vi "Main v1.31.vi"() -> ()   [LabVIEW 2017]
doc: "v0.85:\n- Counts for rejects and total\n\nv0.5:\n\n- Added Reject to Manual Mode\n- Send reject pallet cluster during manual mode\n- Run continuous manual happens only when no error has occured"
uses:
  Controls/Main Tabs v0.1.ctl
  Controls/Auto.ctl
  RT/Controls/Auto Delays.ctl
  RT/Controls/Auto Times.ctl
  support/Controls/General Para.ctl
  Controls/UI Data.ctl
  support/Controls/Auto Stats.ctl
  Controls/Logging FGV.ctl
  support/Message Queue/Enqueue Message (Single).vi
  GV/Maintenance GV.vi
  <vilib>/Utility/error.llb/Error Cluster From Error Code.vi
  <vilib>/ErrorRing/Error Ring.xnode
  support/Message Queue/Message Queue.lvlib
  support/User Event - Stop/User Event - Stop.lvlib
panel:
  in  "General Para 2":T1={"Max. Cons."=5.0, "Offset 1"=0.0, "Offset 2"=0.0, "Offset 3"=0.0, "Offset 4"=0.0} caption="General Para"
  in  "Auto Para 2":T2={"Agitator Delays"=[250, 350], "TF Delays"=[700, 800, 2], "Insertion Delays"=[100, 500], "Cutting Delays"=[300, 300, 100], "PF Delays"=[250, 30000], "Measur. Delays"=[500.0, 188.9, 1.0], "Reject Delays"=[500], "BF Delays"=[1000, 1000]}
  out "Shutdown?":bool
  out "Boolean 8":bool
  out "Boolean 7":bool
  out "Boolean 6":bool
  out "Boolean 5":bool
  out "Boolean 4":bool
  out "Boolean 3":bool
  out "Boolean 2":bool
  out "Boolean":bool
  in  "Reject Pallets":T3
  out "Date-Time":string caption="Dip-Tube Assembly Automation (HMI) v1.2"
  out "Main Tab":T4
  in  "All IOs":bool
  in  "Autocycle":T5
  in  "Manual":bool
  in  "Parameters":bool
  in  "Maintenance":bool
  in  "General Para":T1={"Max. Cons."=5.0, "Offset 1"=0.0, "Offset 2"=0.0, "Offset 3"=0.0, "Offset 4"=0.0} {"Offset 4" format="%.2f"; "Offset 3" format="%.2f"; "Offset 2" format="%.2f"; "Offset 1" format="%.2f"}
  in  "BF Para":cluster{"Delay 1":u32, "Delay 2":u32}={"Delay 1"=1000, "Delay 2"=1000}
  in  "Reject Para":cluster{"Delay":u32}={"Delay"=400}
  in  "Meas. Para":T6={"Delay"=500.0, "Mean Length"=188.9, "Tolerance"=1.0}
  in  "PF Para":cluster{"Delay":u32, "Timeout":u32}={"Delay"=1000, "Timeout"=1000}
  in  "Tube Feeder Para":T7={"Delay"=400, "Delay 2"=250, "Max Attempts"=250}
  in  "Cutting Para":T8={"Delay"=400, "Delay 2"=250, "Delay 3"=250}
  in  "Agitator Para":cluster{"Delay":u32, "Timeout":u32}={"Delay"=400, "Timeout"=250}
  in  "Insertion Para":cluster{"Delay 1":u32, "Delay 2":u32}={"Delay 1"=1000, "Delay 2"=1000}
  in  "Save Para":bool
  in  "Home Para":bool
  out "OEE":dbl format="%#.1f"
  out "QUA":dbl=100.0 min=0.0 max=100.0 step=0.1
  in  "Ideal Time":dbl=2.0 min=0.0 max=100.0 step=0.1
  in  "AVL":dbl=100.0 min=0.0 max=100.0 step=0.1
  out "Rejects 2":u32 caption="Rejects"
  in  "Reset MCount":bool
  in  "Enable BF?":bool
  in  "Enable Agitate?":bool
  in  "Enable Reject?":bool
  in  "Toggle Motor":bool
  in  "Continuous?":bool
  in  "Enable Measure?":bool
  in  "Enable Index?":bool
  in  "Enable PF?":bool
  in  "Manual Para":T2={"Agitator Delays"=[400, 250], "TF Delays"=[700, 800, 2], "Insertion Delays"=[100, 500], "Cutting Delays"=[300, 300, 100], "PF Delays"=[250, 30000], "Measur. Delays"=[500.0, 188.9, 1.0], "Reject Delays"=[500], "BF Delays"=[1000, 1000]}
  in  "Enable Cutting?":bool
  in  "Enable Insertion?":bool
  in  "Run Manual":bool
  in  "Enable TF?":bool
  in  "Home Manual":bool
  out "Status 2":T10
  out "Measurements":T11 {"Height 1" format="%#.2f"; "Height 2" format="%#.2f"; "Height 3" format="%#.2f"; "Height 4" format="%#.2f"}
  out "Output Count":u32 caption="Output\nCount"
  out "PRF":dbl=100.0 min=0.0 max=100.0 step=0.1
  in  "End Cycle":bool
  out "Statuses":string[][](table)
  in  "All IO":bool
  in  "Stats":bool
  in  "Home AC":bool
  out "Status":string
  out "Good":u32 format="%06.0f"
  out "Cycle Time":dbl format="%0.2f"
  out "Rejects":u32 format="%06.0f"
  out "Total Count 2":u32 caption="Total Count"
  out "Avg. Time":dbl caption="Avg. Cycle Time (s)" format="%#.3f"
  out "Output Chart":T12(graph)
  out "Reject Count":u32
  out "Good Count":u32
  out "Total Time":dbl caption="Effective Cycle Time (s)" format="%#.3f"
  out "Time Chart":T13(graph)
  out "OEE Chart":T14(graph)
  out "Timestamp":string caption="Date & Timestamp"
  out "Latest Measure.":T15 caption="Latest Measurements" {"Length 1 (mm)" format="%#.2f"}
  out "Auto Times":T9
  in  "Back Stats":bool
  out "OEE 2":T14 caption="Latest Measurements" {"AVL" format="%#.1f"; "PRF" format="%#.1f"; "QUA" format="%#.1f"; "OEE" format="%#.1f"}
  out "Measurement Chart":T16(graph)
  in  "Home IOs":bool
  in  "Back IO":bool
  out "IAS 4":dbl format="%#.3f"
  out "IAS 3":dbl format="%#.3f"
  out "IAS 2":dbl format="%#.3f"
  out "IAS 1":dbl format="%#.3f"
  out "DI 1":T17
  out "DI 2":T18
  out "DO 1":T19
  in  "Exit":bool
  in  "Shutdown":bool
  # "HARMONY VISION DIP-TUBE ASSEMBLY AUTOMATION"
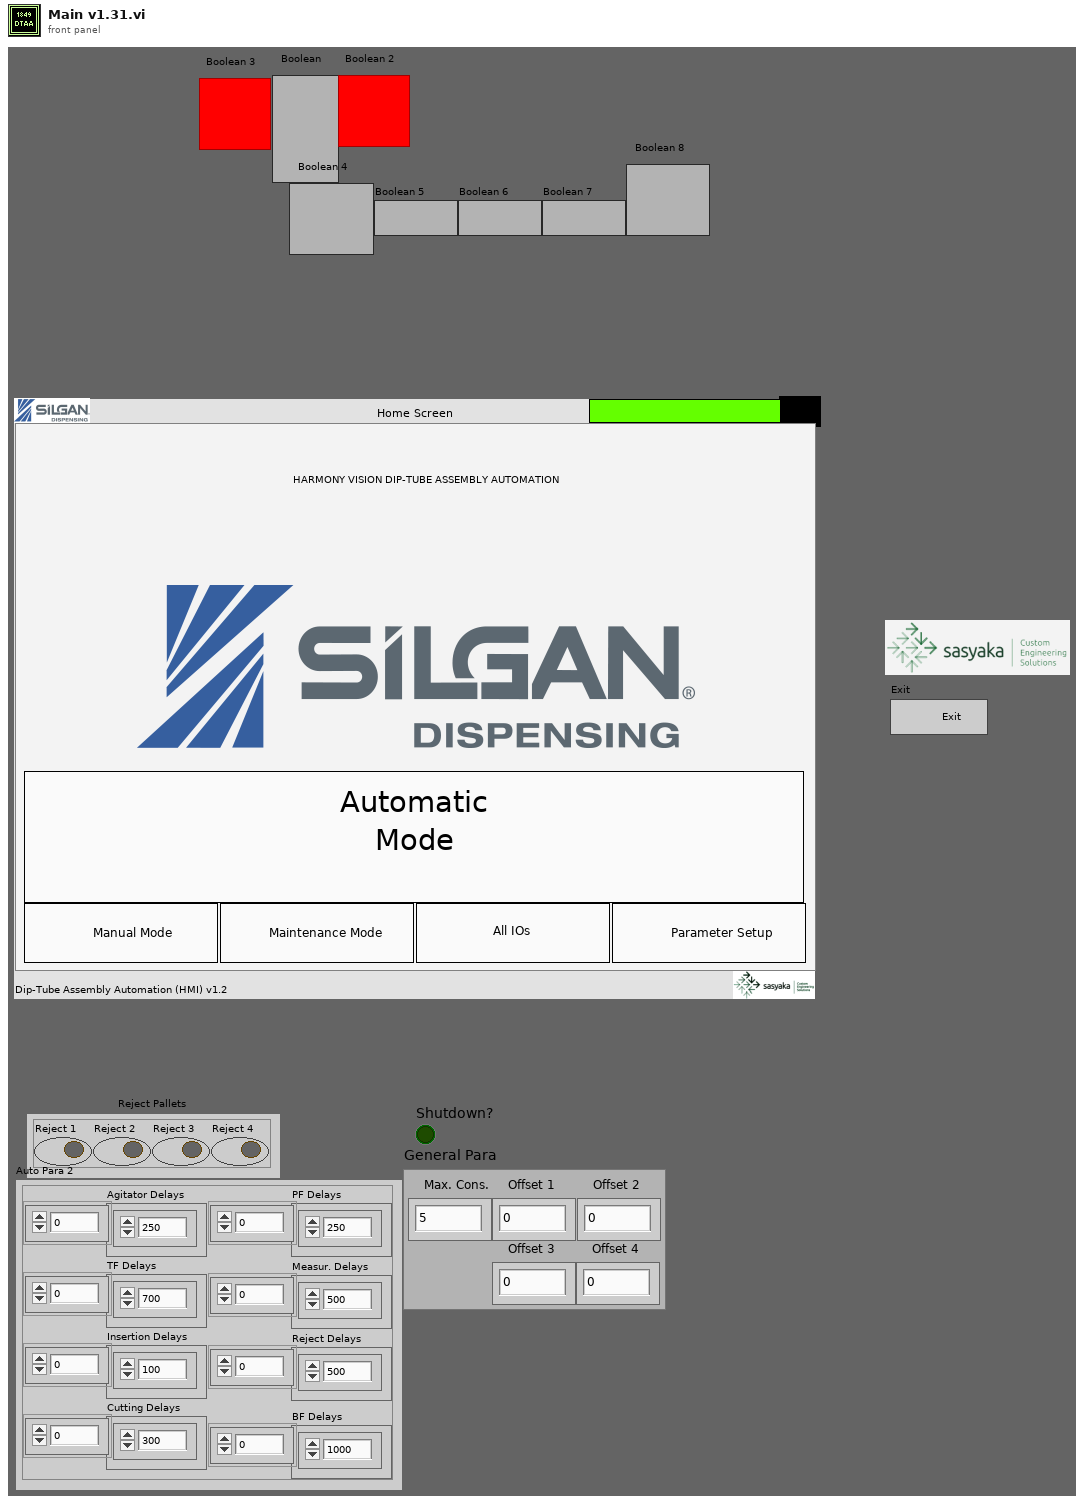
[diagram p1: front panel]
types:
  T1 = typedef "General Para.ctl" = cluster{"Max. Cons.":dbl, "Offset 1":dbl, "Offset 2":dbl, "Offset 3":dbl, "Offset 4":dbl}
  T2 = typedef "Auto Delays.ctl" = cluster{"Agitator Delays":u32[], "TF Delays":u32[], "Insertion Delays":u32[], "Cutting Delays":u32[], "PF Delays":u32[], "Measur. Delays":dbl[], "Reject Delays":u32[], "BF Delays":u32[]}
  T3 = cluster{"Reject 1":bool, "Reject 2":bool, "Reject 3":bool, "Reject 4":bool}
  T4 = typedef "Main Tabs v0.1.ctl" = enum32{"Home Screen", "Parameter Setup", "Manual Mode", "Autocycle", "Autocycle Statistics", "Autocycle IOs"}
  T5 = typedef "Auto.ctl" = bool
  T6 = cluster{"Delay":dbl, "Mean Length":dbl, "Tolerance":dbl}
  T7 = cluster{"Delay":u32, "Delay 2":u32, "Max Attempts":u32}
  T8 = cluster{"Delay":u32, "Delay 2":u32, "Delay 3":u32}
  T9 = typedef "Auto Times.ctl" = cluster{"Index Time":u32, "TF Time":u32, "Insertion Time":u32, "Cutting Time":u32, "PF Time":u32, "Meas. Time":u32, "Reject Time":u32}
  T10 = cluster{"Auto Times":T9, "error out":errorcluster}
  T11 = cluster{"Height 1":dbl, "Height 2":dbl, "Height 3":dbl, "Height 4":dbl}
  T12 = cluster{"OutputCount":u32, "Numeric Control":u32}
  T13 = cluster{"Index":dbl, "TF":dbl, "Insert":dbl, "Cutting":dbl, "PF":dbl, "Measure.":dbl, "Reject":dbl}
  T14 = cluster{"AVL":dbl, "PRF":dbl, "QUA":dbl, "OEE":dbl}
  T15 = cluster{"Length 1 (mm)":dbl, "Pallet 2 (mm)":dbl, "Pallet 3 (mm)":dbl, "Pallet 4 (mm)":dbl}
  T16 = cluster{"1":dbl, "2":dbl, "3":dbl, "4":dbl, "4":dbl, "4":dbl}
  T17 = cluster{"Machine_ON":bool, "E_stop ":bool, "SW_Pressure":bool, "SW_Start ":bool, "SW_Reset":bool, "SW_Stop":bool, "SW_Door":bool, "RS_Index_Rotary_CW":bool, "RS_Index_Rotary_CCW":bool, "RS_Index_Stopper _Rear":bool, "RS_Index_Output_Separator_Rear":bool, "PES_Index_Pallet_Sensor":bool, "PES_Index_Output_Part Sensor":bool, "ICS_BF_Low_Level_1":bool, "ICS_BF_Low_Level_2":bool, "ICS_BF_Pump_CNVR_Full_1":bool, "ICS_BF_Pump_CNVR_Full_2":bool, "ICS_BF_Pump_CNVR_Full_3":bool, "ICS_BF_Pump_CNVR_Full_4":bool, "PES_PC_Pump Presence_1":bool, "PES_PC_Pump Presence_2":bool, "PES_PC_Pump Presence_3":bool, "PES_PC_Pump Presence_4":bool, "RS_PC_Gating_Front":bool, "PES_Pump_Interference":bool, "PES_TF_Low_Level":bool, "PES_Tube Presence_1":bool, "PES_Tube Presence_2":bool, "PES_Tube Presence_3":bool, "PES_Tube Presence_4":bool, "DI1.30":bool, "DI1.31":bool}
  T18 = cluster{"RS_Agitatator_1_Rear ":bool, "RS_Agitatator_2_Rear ":bool, "RS_TF_Gating CYL_Rear":bool, "RS_Insertion_1_Rear":bool, "RS_Insertion_1_Front":bool, "RS_Insertion _2_Rear":bool, "RS_Insertion _2_Front":bool, "RS_Insertion _3_Rear":bool, "RS_Insertion _3_Front":bool, "RS_Insertion _4_Rear":bool, "RS_Insertion _4_Front":bool, "RS_Insertion_Clamp_Rear":bool, "RS_Cutting_Rear":bool, "RS_Cutting_Clamp _Rear":bool, "RS_Measurement_1_Rear":bool, "RS_Measurement_2_Rear":bool, "RS_Measurement_3_Rear":bool, "RS_Measurement_4_Rear":bool, "DI2.18":bool, "RS_Rejection_1_Rear":bool, "RS_Rejection_2_Rear":bool, "RS_Rejection_3_Rear":bool, "RS_Rejection_4_Rear":bool, "DI2.23":bool, "DI2.24":bool, "DI2.25":bool, "DI2.26":bool, "DI2.27":bool, "DI2.28":bool, "DI2.29":bool, "DI2.30":bool, "DI2.31":bool}
  T19 = cluster{"TL_Red":bool, "TL_Orange":bool, "TL_Green":bool, "TL_Buzzer":bool, "SOL_Index_Rotary_CW":bool, "SOL_Index_Rotary_CCW":bool, "SOL_Index_Stopper_Rear":bool, "SOL_OutputSeparator_Rear":bool, "Bowl  Feeder_ ON 1":bool, "Pump_CNVR_Motor _ON":bool, "SOL_PC_Gating_CYL_Rear":bool, "SOL_Tube_Feed_Agitatator":bool, "SOL_Tube_Feed_Gating_CYL":bool, "SOL_Insertion _CYL":bool, "SOL_Insertion_Clamp_CYL":bool, "SOL_Cutting_CYL":bool, "SOL_Cutting_Clamp_CYL":bool, "SOL_Insertion_Air_Nozzle":bool, "SOL_Measurement_CYL":bool, "DO1.19":bool, "SOL_Rejection CYL_1":bool, "SOL_Rejection CYL_2":bool, "SOL_Rejection CYL_3":bool, "SOL_Rejection CYL_4":bool, "Bowl  Feeder_ ON 2":bool, "SOL_BF_BlowerON":bool, "SOL_BF1_Track1":bool, "SOL_BF1_Track2":bool, "SOL_BF2_Track1":bool, "SOL_BF2_Track2":bool, "DO1.30":bool, "DO1.31":bool}
  T20 = typedef "UI Data.ctl" = cluster{"Main Tab":refnum<vi>}
  T21 = typedef "Message Queue.lvlib/All Message Queues.ctl" = cluster{"UI":refnum<queue>}
  T22 = enum8{"Enabled", "Disabled", "Disabled and Grayed Out"}
  T23 = cluster{"Array":string[][], "Machine Status":string}
  T24 = typedef "Logging FGV.ctl" = enum16{"Start Shift", "Log Index", "Read Shift", "Close Shift"}
  T25 = typedef "Auto Stats.ctl" = cluster{"Time-Stamp":timestamp, "Auto Times":T9, "Measurements":cluster{"1":dbl, "2":dbl, "3":dbl, "4":dbl}, "Outputs":cluster{"Good Parts":u32, "Reject Parts":u32}, "Cycle Time":dbl, "Remarks":string}
  T26 = cluster{"Auto Times":T9, "Results":cluster{"Measurements":cluster{"1":dbl, "2":dbl, "3":dbl, "4":dbl}, "Reject Pallets":cluster{"Reject 1":bool, "Reject 2":bool, "Reject 3":bool, "Reject 4":bool}}, "OutputCount":u32, "error out":errorcluster}
  T27 = enum8{"Information", "Error", "Successful", "Tips"}
  T28 = cluster{"Agitator Delays[0]":u32, "Agitator Delays[1]":u32}
  T29 = cluster{"TF Delays[0]":u32, "TF Delays[1]":u32, "TF Delays[2]":u32}
  T30 = cluster{"Insertion Delays[0]":u32, "Insertion Delays[1]":u32}
  T31 = cluster{"Cutting Delays[0]":u32, "Cutting Delays[1]":u32, "Cutting Delays[2]":u32}
  T32 = cluster{"Measur. Delays[0]":dbl, "Measur. Delays[1]":dbl, "Measur. Delays[2]":dbl}
  T33 = typedef "All Inputs.ctl" = cluster{"DI 1":cluster{"Machine_ON":bool, "E_stop ":bool, "SW_Pressure":bool, "SW_Start ":bool, "SW_Reset":bool, "SW_Stop":bool, "SW_Door":bool, "RS_Index_Rotary_CW":bool, "RS_Index_Rotary_CCW":bool, "RS_Index_Stopper _Rear":bool, "RS_Index_Output_Separator_Rear":bool, "PES_Index_Pallet_Sensor":bool, "PES_Index_Output_Part Sensor":bool, "ICS_BF_Low_Level_1":bool, "ICS_BF_Low_Level_2":bool, "ICS_BF_Pump_CNVR_Full_1":bool, "ICS_BF_Pump_CNVR_Full_2":bool, "ICS_BF_Pump_CNVR_Full_3":bool, "ICS_BF_Pump_CNVR_Full_4":bool, "PES_PC_Pump Presence_1":bool, "PES_PC_Pump Presence_2":bool, "PES_PC_Pump Presence_3":bool, "PES_PC_Pump Presence_4":bool, "RS_PC_Gating_Front":bool, "PES_Pump_Interference":bool, "PES_TF_Low_Level":bool, "PES_Tube Presence_1":bool, "PES_Tube Presence_2":bool, "PES_Tube Presence_3":bool, "PES_Tube Presence_4":bool, "DI1.30":bool, "DI1.31":bool}, "DI 2":cluster{"RS_Agitatator_1_Rear ":bool, "RS_Agitatator_2_Rear ":bool, "RS_TF_Gating CYL_Rear":bool, "RS_Insertion_1_Rear":bool, "RS_Insertion_1_Front":bool, "RS_Insertion _2_Rear":bool, "RS_Insertion _2_Front":bool, "RS_Insertion _3_Rear":bool, "RS_Insertion _3_Front":bool, "RS_Insertion _4_Rear":bool, "RS_Insertion _4_Front":bool, "RS_Insertion_Clamp_Rear":bool, "RS_Cutting_Rear":bool, "RS_Cutting_Clamp _Rear":bool, "RS_Measurement_1_Rear":bool, "RS_Measurement_2_Rear":bool, "RS_Measurement_3_Rear":bool, "RS_Measurement_4_Rear":bool, "RS_Measure_Clamp_Rear":bool, "RS_Rejection_1_Rear":bool, "RS_Rejection_2_Rear":bool, "RS_Rejection_3_Rear":bool, "RS_Rejection_4_Rear":bool, "DI2.23":bool, "DI2.24":bool, "DI2.25":bool, "DI2.26":bool, "DI2.27":bool, "DI2.28":bool, "DI2.29":bool, "DI2.30":bool, "DI2.31":bool}, "IAS 1":dbl, "IAS 2":dbl, "IAS 3":dbl, "IAS 4":dbl, "DO 1":cluster{"TL_Red":bool, "TL_Orange":bool, "TL_Green":bool, "TL_Buzzer":bool, "SOL_Index_Rotary_CW":bool, "SOL_Index_CNVR_Rotary_CCW":bool, "SOL_Index_CNVR_Stopper_Rear":bool, "SOL_Index_CNVR_Output _Separator _Rear":bool, "Bowl  Feeder_ ON 1":bool, "Pump_CNVR_Motor _ON":bool, "SOL_PC_Gating_CYL_Rear":bool, "SOL_Tube_Feed_Agitatator":bool, "SOL_Tube_Feed_Gating_CYL":bool, "SOL_Insertion _CYL":bool, "SOL_Insertion_Clamp_CYL":bool, "SOL_Cutting_CYL":bool, "SOL_Cutting_Clamp_CYL":bool, "SOL_Insertion_Air_Nozzle":bool, "SOL_Measurement_CYL":bool, "DO1.19":bool, "SOL_Rejection CYL_1":bool, "SOL_Rejection CYL_2":bool, "SOL_Rejection CYL_3":bool, "SOL_Rejection CYL_4":bool, "Bowl  Feeder_ ON 2":bool, "SOL_BF_BlowerON":bool, "SOL_BF1_Track1":bool, "SOL_BF1_Track2":bool, "SOL_BF2_Track1":bool, "SOL_BF2_Track2":bool, "DO1.30":bool, "DO1.31":bool}}
  T34 = cluster{"RS_Agitatator_1_Rear ":bool, "RS_Agitatator_2_Rear ":bool, "RS_TF_Gating CYL_Rear":bool, "RS_Insertion_1_Rear":bool, "RS_Insertion_1_Front":bool, "RS_Insertion _2_Rear":bool, "RS_Insertion _2_Front":bool, "RS_Insertion _3_Rear":bool, "RS_Insertion _3_Front":bool, "RS_Insertion _4_Rear":bool, "RS_Insertion _4_Front":bool, "RS_Insertion_Clamp_Rear":bool, "RS_Cutting_Rear":bool, "RS_Cutting_Clamp _Rear":bool, "RS_Measurement_1_Rear":bool, "RS_Measurement_2_Rear":bool, "RS_Measurement_3_Rear":bool, "RS_Measurement_4_Rear":bool, "RS_Measure_Clamp_Rear":bool, "RS_Rejection_1_Rear":bool, "RS_Rejection_2_Rear":bool, "RS_Rejection_3_Rear":bool, "RS_Rejection_4_Rear":bool, "DI2.23":bool, "DI2.24":bool, "DI2.25":bool, "DI2.26":bool, "DI2.27":bool, "DI2.28":bool, "DI2.29":bool, "DI2.30":bool, "DI2.31":bool}
  T35 = cluster{"TL_Red":bool, "TL_Orange":bool, "TL_Green":bool, "TL_Buzzer":bool, "SOL_Index_Rotary_CW":bool, "SOL_Index_CNVR_Rotary_CCW":bool, "SOL_Index_CNVR_Stopper_Rear":bool, "SOL_Index_CNVR_Output _Separator _Rear":bool, "Bowl  Feeder_ ON 1":bool, "Pump_CNVR_Motor _ON":bool, "SOL_PC_Gating_CYL_Rear":bool, "SOL_Tube_Feed_Agitatator":bool, "SOL_Tube_Feed_Gating_CYL":bool, "SOL_Insertion _CYL":bool, "SOL_Insertion_Clamp_CYL":bool, "SOL_Cutting_CYL":bool, "SOL_Cutting_Clamp_CYL":bool, "SOL_Insertion_Air_Nozzle":bool, "SOL_Measurement_CYL":bool, "DO1.19":bool, "SOL_Rejection CYL_1":bool, "SOL_Rejection CYL_2":bool, "SOL_Rejection CYL_3":bool, "SOL_Rejection CYL_4":bool, "Bowl  Feeder_ ON 2":bool, "SOL_BF_BlowerON":bool, "SOL_BF1_Track1":bool, "SOL_BF1_Track2":bool, "SOL_BF2_Track1":bool, "SOL_BF2_Track2":bool, "DO1.30":bool, "DO1.31":bool}
  T36 = cluster{"Manual Para":T2, "Reject Pallets":cluster{"Reject 1":bool, "Reject 2":bool, "Reject 3":bool, "Reject 4":bool}}
  T37 = cluster{"Measurements":cluster{"1":dbl, "2":dbl, "3":dbl, "4":dbl}, "Reject Pallets":cluster{"Reject 1":bool, "Reject 2":bool, "Reject 3":bool, "Reject 4":bool}}
  T38 = cluster{"Reject Pallets":cluster{"Reject 1":bool, "Reject 2":bool, "Reject 3":bool, "Reject 4":bool}, "Measurements":cluster{"1":dbl, "2":dbl, "3":dbl, "4":dbl}}
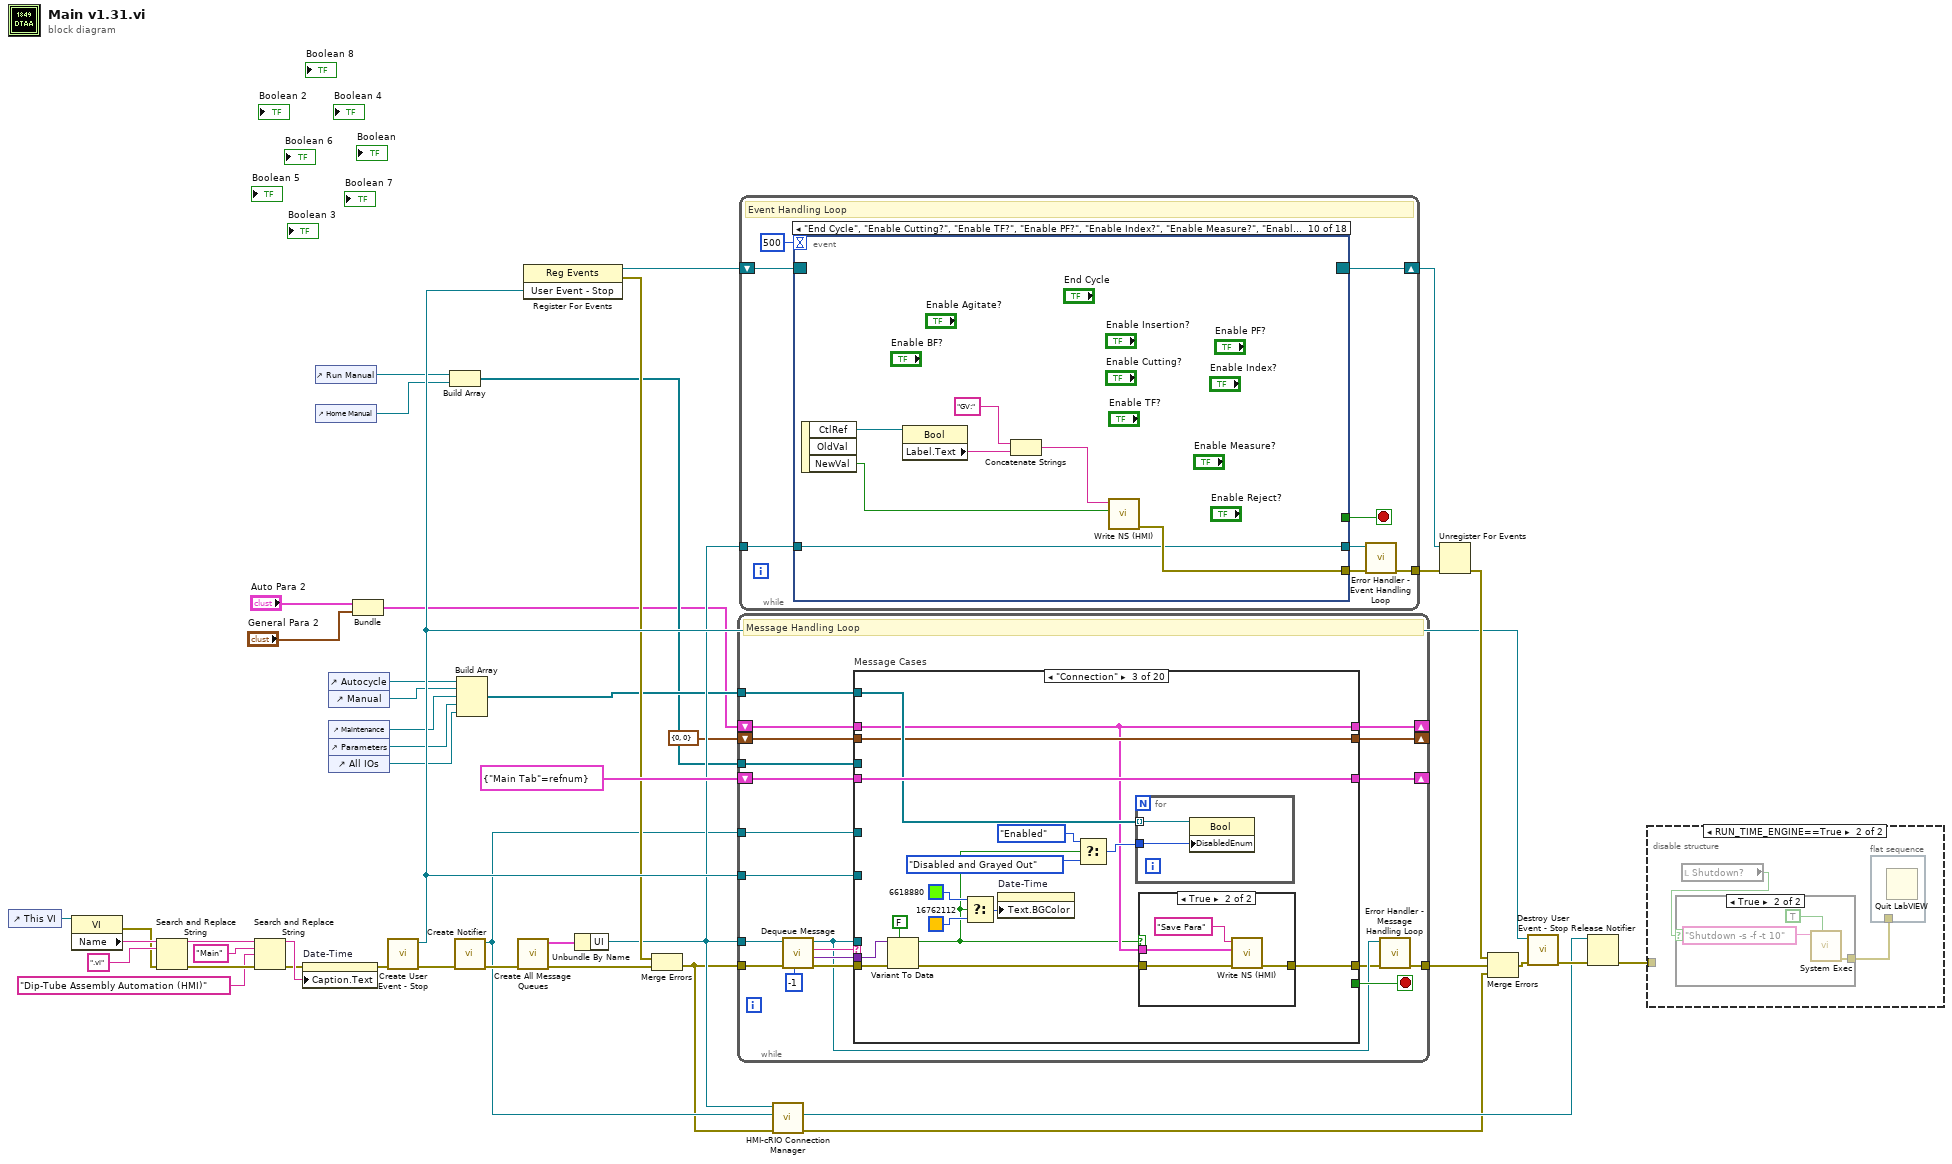
[diagram p0: block diagram]
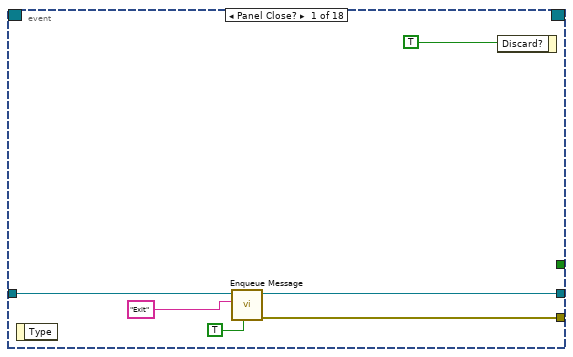
[diagram p2: hidden frame]
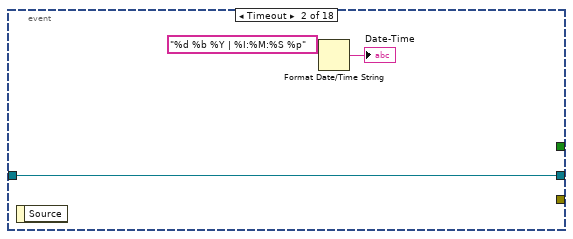
[diagram p3: hidden frame]
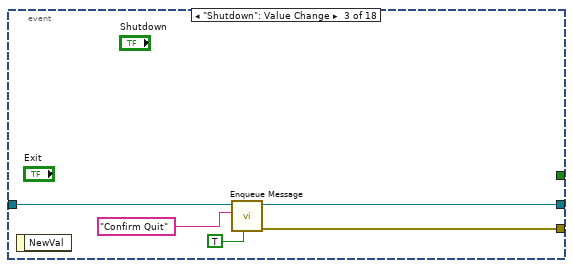
[diagram p4: hidden frame]
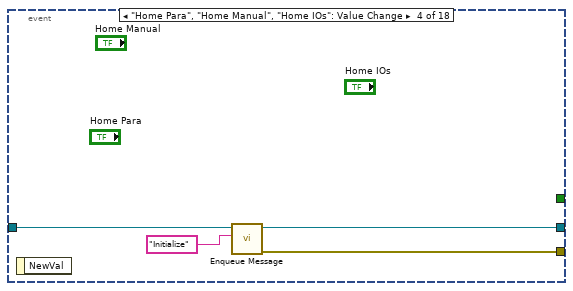
[diagram p5: hidden frame]
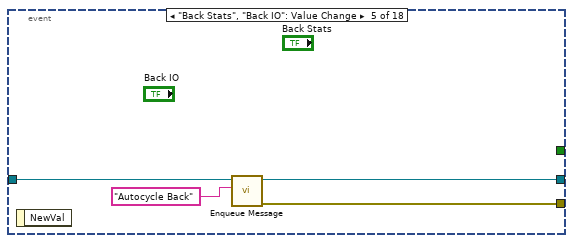
[diagram p6: hidden frame]
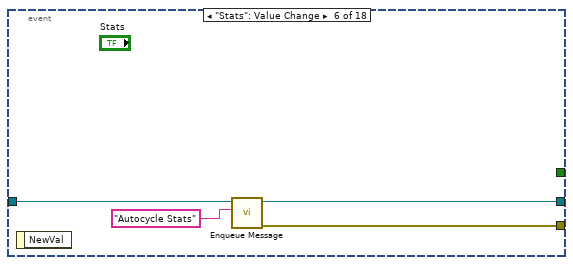
[diagram p7: hidden frame]
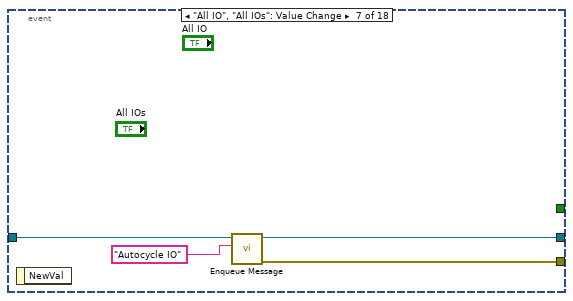
[diagram p8: hidden frame]
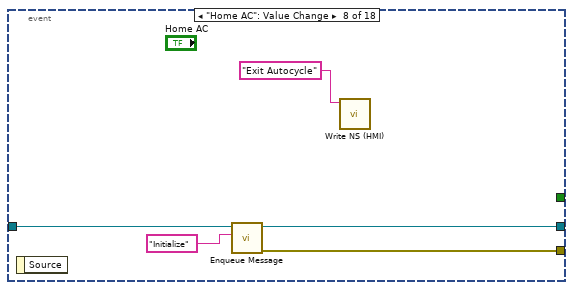
[diagram p9: hidden frame]
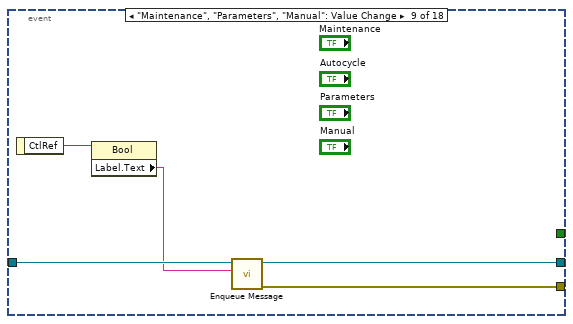
[diagram p10: hidden frame]
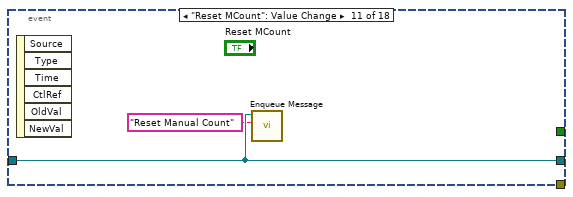
[diagram p11: hidden frame]
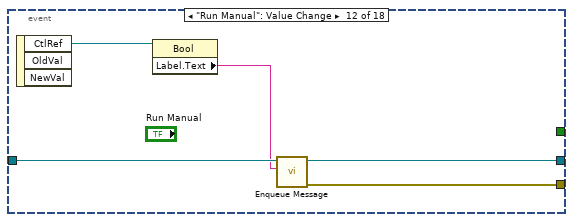
[diagram p12: hidden frame]
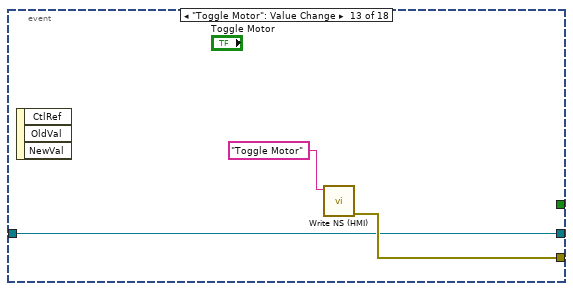
[diagram p13: hidden frame]
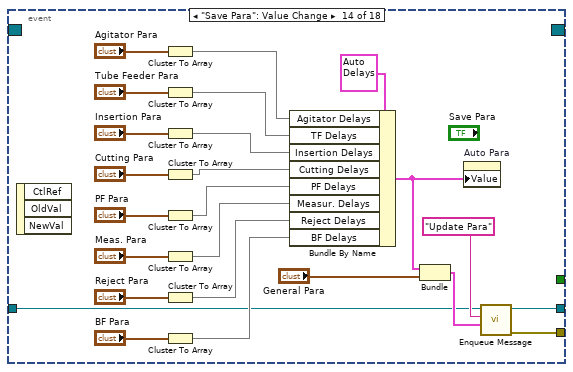
[diagram p14: hidden frame]
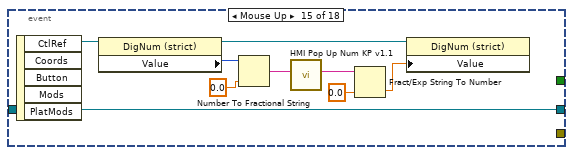
[diagram p15: hidden frame]
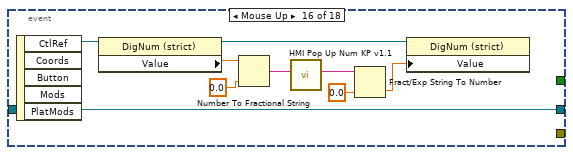
[diagram p16: hidden frame]
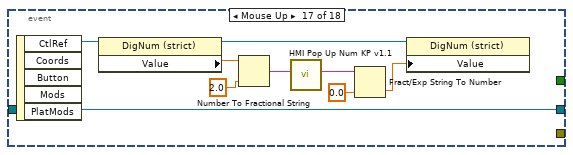
[diagram p17: hidden frame]
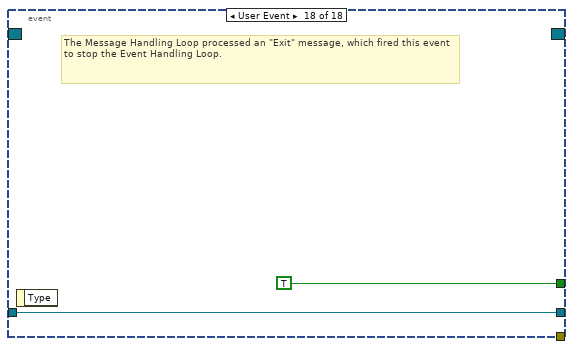
[diagram p18: hidden frame]
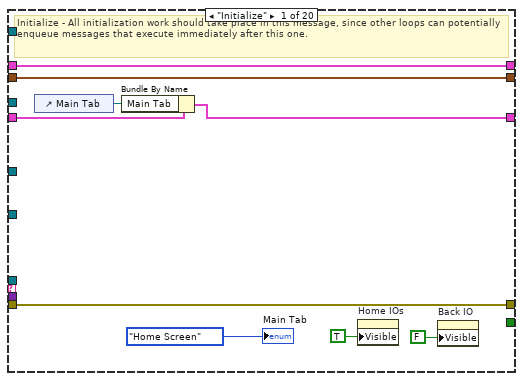
[diagram p19: hidden frame]
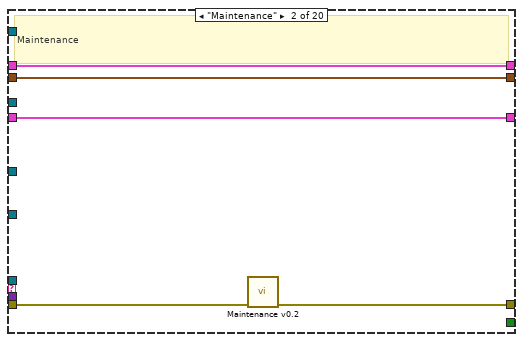
[diagram p20: hidden frame]
diagram:
  n1 = control-ref of="This VI"() -> (w15:refnum<vi>)
  n2 = property class="VI"(reference=w15) -> (error out=w14:errorcluster, "Name"=w21:string)  [unwired: 1 in, 1 out]
  n3 = Search and Replace String(input string=w21, search string=".vi", error in=w14) -> (result string=w19:string, error out=w18:errorcluster)  [unwired: 5 in, 2 out]
  n4 = Search and Replace String(input string=w19, search string="Main", replace string="Dip-Tube Assembly Automation (HMI)" ("replace string (\"\")"), error in=w18) -> (result string=w13:string, error out=w12:errorcluster)  [unwired: 4 in, 2 out]
  n5 = property on="Date-Time" class="Str"(error in=w12, "Caption.Text"=w13) -> (error out=w11:errorcluster)  [unwired: 1 in, 1 out]
  n6 = control-ref of="Run Manual"() -> (w10:refnum<vi>)
  n7 = control-ref of="Home Manual"() -> (w9:refnum<vi>)
  n8 = control-ref of="Autocycle"() -> (w26:refnum<vi>)
  n9 = control-ref of="Manual"() -> (w25:refnum<vi>)
  n10 = control-ref of="Maintenance"() -> (w24:refnum<vi>)
  n11 = control-ref of="Parameters"() -> (w23:refnum<vi>)
  n12 = control-ref of="All IOs"() -> (w4:refnum<vi>)
  n13 = Bundle("Auto Para 2"="Auto Para 2", "General Para 2"="General Para 2") -> (w1:cluster{"Auto Para 2":T2, "General Para 2":T1})  [unwired: 1 in]
  n14 = call "Create User Event - Stop.vi"("error in (no error)"=w11) -> ("error out"=w32:errorcluster, "User Event - Stop"=w35:refnum<user-event>)  [unwired: 9 in]
  n15 = Build Array(w10, w9) -> (w8:refnum<vi>[])
  n16 = call "Create Notifier.vi"("error in (no error)"=w32) -> ("error out"=w31:errorcluster, "notifier out"=w6:refnum<notifier>)  [unwired: 9 in]
  n17 = Build Array(w26, w25, w24, w23, w4) -> (w22:refnum<vi>[])
  n18 = call "Create All Message Queues.vi"("error in (no error)"=w31) -> ("error out"=w44:errorcluster, "Message Queues out"=w43:T21)  [unwired: 9 in]
  n19 = register-events(w35) -> (reference out=w36:refnum<event-registration>, error out=w34:errorcluster)  [unwired: 2 in]
  n20 = Unbundle By Name(w43) -> ("UI"=w33:refnum<queue>)
  n21 = Merge Errors(w34, w44) -> (w5:errorcluster)
  n22 = while {
    tunnel: w33 -> [w57]
    shift-right: [w64] -> _
    shift-left: T20 {"Main Tab"=refnum} ("Data Cluster") -> [w47]
    tunnel: w35 -> [w62]
    tunnel: w5 -> [w61]
    tunnel: [w55] -> w42
    tunnel: w6 -> [w52]
    tunnel: w22 -> [w51]
    tunnel: w8 -> [w50]
    shift-right: [w48] -> _
    shift-left: cluster{"OutputCount":u32, "RejectCount":u32} {"OutputCount"=0, "RejectCount"=0} -> [w49]
    shift-right: [w45] -> _
    shift-left: w1 -> [w46]
    stop <- w63 stop-if-true
    # "Message Handling Loop"
    n23 = call "Dequeue Message.vi"("timeout"=-1, "error in (no error)"=w61, "Message Queue"=w57) -> ("error out"=w60:errorcluster, "Message Data"=w58:variant, "Message"=w59:string, "dup Message Queue"=w56:refnum<queue>)  [unwired: 5 in]
    n24 = case "Message Cases" shown="\"Connection\"" w59 {
      selector: w59 -> [_ _ _ _ _ _ _ _ _ _ _ _ _ _ _ _ _ _ _ w379]
      tunnel: w56 -> [_ _ _ _ _ _ _ _ _ w185 w194 _ _ _ w298 _ _ w350 w376 _]
      tunnel: w60 -> [w73 w77 w92 w121 w132 w149 w157 w173 w179 w187 w202 w231 w262 w273 w306 w317 w341 w354 w369 _]
      tunnel: [w73 w76 w81 w121 w127 w149 w156 w173 w179 w186 w201 w232 w263 w275 w297 w317 w336 w352 w372 w380] -> w54
      tunnel: w47 -> [w72 w78 w94 w125 w134 w148 w153 w177 w183 w192 w199 w233 w264 w276 w307 w316 w340 w353 w375 w381]
      tunnel: [w71 w78 w94 w125 w134 w148 w153 w177 w183 w192 w199 w233 w264 w276 w307 w316 w340 w353 w375 w381] -> w64
      tunnel: [_ _ _ _ _ _ _ _ _ _ _ _ _ _ _ _ _ _ TRUE _] -> w63
      tunnel: w58 -> [_ _ w91 _ w131 _ _ _ _ _ _ w230 w261 _ w305 _ w339 _ w366 _]
      tunnel: w62 -> [_ _ _ _ _ _ _ _ _ _ _ _ _ _ _ _ _ _ w371 _]
      tunnel: w52 -> [_ _ _ _ _ _ _ _ _ _ _ _ _ _ _ _ _ _ w365 _]
      tunnel: w51 -> [_ _ w87 _ _ _ _ _ _ _ _ _ _ _ _ _ _ _ _ _]
      tunnel: w50 -> [_ _ _ _ _ _ _ _ _ _ _ _ _ w270 w303 _ _ _ _ _]
      tunnel: w49 -> [w68 w75 w83 w122 w133 w137 w158 w174 w180 w189 w203 w228 w259 w266 w296 _ w335 w349 w362 w378]
      tunnel: [w68 w75 w83 w122 w133 w137 w158 w174 w180 w189 w203 w228 w259 w266 w291 cluster{"OutputCount":u32, "RejectCount":u32} {"OutputCount"=0, "RejectCount"=0} w335 w349 w362 w378] -> w48
      tunnel: w46 -> [w65 w74 w80 w102 _ w136 w152 w172 w178 w184 w193 w217 w246 w265 w279 w313 w318 w342 w361 w377]
      tunnel: [w65 w74 w80 w102 w126 w136 w152 w172 w178 w184 w193 w217 w246 w265 w279 w313 w318 w342 w361 w377] -> w45
      frame "Initialize" {
        # "Initialize - All initialization work should take place in this message, since other loops can potentially enqueue messages that execute immediately after this one."
        n25 = control-ref of="Main Tab"() -> (w70:refnum<vi>)
        n26 = Bundle By Name(cluster=w72, "Main Tab"=w70) -> (w71:T20)
        n27 = property on="Home IOs" class="Bool"("Visible"=TRUE) -> ()  [unwired: 2 in, 2 out]
        n28 = property on="Back IO" class="Bool"("Visible"=FALSE) -> ()  [unwired: 2 in, 2 out]
        "Main Tab" <- Main_Tabs_v0.1."Home Screen" ("Main Tab")
      }
      frame "Maintenance" {
        # "Maintenance"
        n29 = call "Maintenance v0.2.vi"("Error In"=w77) -> ("Error out"=w76:errorcluster)  [unwired: 10 in]
      }
      frame "Connection" {
        n30 = Variant To Data(error in=w92, type=FALSE, Variant=w91) -> (data=w79:bool, error out=w82:errorcluster)
        n31 = Select(t=u32 6618880 ("Text.Text Colors:BG Color"), s=w79, f=u32 16762112 ("Text.Text Colors:BG Color")) -> (s? t:f=w88:u32)
        n32 = property on="Date-Time" class="Str"("Text.BGColor"=w88) -> ()  [unwired: 2 in, 2 out]
        n33 = Select(t=T22."Enabled" ("Disabled"), s=w79, f=T22."Disabled and Grayed Out") -> (s? t:f=w85:T22)
        n34 = for {
          tunnel: w87 -> [w101] mode=indexing
          tunnel: w85 -> [w100]
          n35 = property class="Bool"(reference=w101, "DisabledEnum"=w100) -> ()  [unwired: 1 in, 2 out]
        }
        n36 = case shown="True" w79 {
          tunnel: w82 -> [w95 w98]
          tunnel: [w95 w97] -> w81
          tunnel: w80 -> [_ w96]
          frame False {
          }
          frame True {
            n37 = call "Write NS (HMI).vi"("error in (no error)"=w98, "Message Data"=w96, "Message"="Save Para") -> ("error out"=w97:errorcluster)  [unwired: 8 in]
          }
        }
      }
      frame "Parameters" {
        # "Parameters"
        n38 = Unbundle(w102) -> ("Auto Para 2"=w104:T2, "General Para 2"=w103:T1)
        n39 = Unbundle By Name(w125) -> ("Main Tab"=w124:refnum<vi>)
        n40 = property on="General Para" class="Clust (strict)"("Value"=w103) -> ()  [unwired: 2 in, 2 out]
        n41 = Unbundle(w104) -> ("Agitator Delays"=w120:u32[], "TF Delays"=w119:u32[], "Insertion Delays"=w118:u32[], "Cutting Delays"=w117:u32[], "PF Delays"=w116:u32[], "Measur. Delays"=w115:dbl[], "Reject Delays"=w114:u32[], "BF Delays"=w113:u32[])
        n42 = property class="TabCtl"(reference=w124, "Value"=Main_Tabs_v0.1."Parameter Setup" ("Main Tab")) -> ()  [unwired: 1 in, 2 out]
        n43 = Array To Cluster(array=w120) -> (cluster=w112:T28)
        n44 = Array To Cluster(array=w119) -> (cluster=w111:T29)
        n45 = Array To Cluster(array=w118) -> (cluster=w110:T30)
        n46 = Array To Cluster(array=w117) -> (cluster=w109:T31)
        n47 = Array To Cluster(array=w116) -> (cluster=w108:cluster{"PF Delays[0]":u32, "PF Delays[1]":u32})
        n48 = Array To Cluster(array=w115) -> (cluster=w107:T32)
        n49 = Array To Cluster(array=w114) -> (cluster=w106:cluster{"Reject Delays[0]":u32})
        n50 = Array To Cluster(array=w113) -> (cluster=w105:cluster{"BF Delays[0]":u32, "BF Delays[1]":u32})
        n51 = property on="Agitator Para" class="Clust (strict)"("Value"=w112) -> ()  [unwired: 2 in, 2 out]
        n52 = property on="Tube Feeder Para" class="Clust (strict)"("Value"=w111) -> ()  [unwired: 2 in, 2 out]
        n53 = property on="Insertion Para" class="Clust (strict)"("Value"=w110) -> ()  [unwired: 2 in, 2 out]
        n54 = property on="Cutting Para" class="Clust (strict)"("Value"=w109) -> ()  [unwired: 2 in, 2 out]
        n55 = property on="PF Para" class="Clust (strict)"("Value"=w108) -> ()  [unwired: 2 in, 2 out]
        n56 = property on="Meas. Para" class="Clust (strict)"("Value"=w107) -> ()  [unwired: 2 in, 2 out]
        n57 = property on="Reject Para" class="Clust (strict)"("Value"=w106) -> ()  [unwired: 2 in, 2 out]
        n58 = property on="BF Para" class="Clust (strict)"("Value"=w105) -> ()  [unwired: 2 in, 2 out]
      }
      frame "Update Para" {
        # "Parameters"
        n59 = Variant To Data(error in=w132, type=cluster{"Auto Para":T2, "General Para":T1} {"Auto Para"={"Agitator Delays"=[], "TF Delays"=[], "Insertion Delays"=[], "Cutting Delays"=[], "PF Delays"=[], "Measur. Delays"=[], "Reject Delays"=[], "BF Delays"=[]}, "General Para"={"Max. Cons."=0.0, "Offset 1"=0.0, "Offset 2"=0.0, "Offset 3"=0.0, "Offset 4"=0.0}} ("cluster"), Variant=w131) -> (data=w126:cluster{"Auto Para":T2, "General Para":T1}, error out=w128:errorcluster)
        n60 = call "Write NS (HMI).vi"("error in (no error)"=w128, "Message Data"=w126, "Message"="Save Para") -> ("error out"=w127:errorcluster)  [unwired: 8 in]
      }
      frame "Manual" {
        # "Parameters"
        n61 = control-ref of="Enable Index?"() -> (w145:refnum<vi>)
        n62 = control-ref of="Enable PF?"() -> (w144:refnum<vi>)
        n63 = control-ref of="Enable Cutting?"() -> (w143:refnum<vi>)
        n64 = control-ref of="Enable Insertion?"() -> (w142:refnum<vi>)
        n65 = control-ref of="Enable TF?"() -> (w141:refnum<vi>)
        n66 = control-ref of="Enable Measure?"() -> (w139:refnum<vi>)
        n67 = Unbundle By Name(w136) -> ("Auto Para 2"=w135:T2)
        n68 = control-ref of="Enable Reject?"() -> (w138:refnum<vi>)
        n69 = Build Array(w145, w144, w143, w142, w141, w139, w138) -> (w140:refnum<vi>[])
        n70 = property on="Auto Para" class="Clust (strict)"("Value"=w135) -> ()  [unwired: 2 in, 2 out]
        n71 = for {
          tunnel: w140 -> [w151] mode=indexing
          n72 = property class="Bool (strict)"(reference=w151, "Val(Sgnl)"=FALSE ("Value (Signaling)")) -> ()  [unwired: 1 in, 2 out]
        }
        n73 = Unbundle By Name(w148) -> ("Main Tab"=w147:refnum<vi>)
        n74 = property class="TabCtl"(reference=w147, "Value"=Main_Tabs_v0.1."Manual Mode" ("Main Tab")) -> ()  [unwired: 1 in, 2 out]
      }
      frame "Autocycle" {
        # "Parameters"
        n75 = call "Select Model v0.1.vi"() -> ("Cancel out"=w154:bool, "Model out"=w155:string)  [unwired: 9 in, 1 out]
        n76 = case shown="False" w154 {
          tunnel: w157 -> [w162 w171]
          tunnel: [w169 w171] -> w156
          tunnel: w155 -> [w168 _]
          tunnel: w153 -> [w165 _]
          tunnel: w152 -> [w159 _]
          frame False {
            n77 = Unbundle By Name(w165) -> ("Main Tab"=w167:refnum<vi>)
            n78 = call "Write NS (HMI).vi"("error in (no error)"=w162, "Message Data"=w159, "Message"="Save Para") -> ("error out"=w161:errorcluster)  [unwired: 8 in]
            n79 = property class="TabCtl"(reference=w167, "Value"=Main_Tabs_v0.1."Autocycle" ("Main Tab")) -> ()  [unwired: 1 in, 2 out]
            n80 = call "Write NS (HMI).vi"("error in (no error)"=w161, "Message Data"=w168, "Message"="Autocycle") -> ("error out"=w169:errorcluster)  [unwired: 8 in]
            n81 = property on="Home IOs" class="Bool"("Visible"=FALSE) -> ()  [unwired: 2 in, 2 out]
            n82 = property on="Back IO" class="Bool"("Visible"=TRUE) -> ()  [unwired: 2 in, 2 out]
          }
          frame True {
          }
        }
      }
      frame "Autocycle Back" {
        # "Parameters"
        n83 = Unbundle By Name(w177) -> ("Main Tab"=w176:refnum<vi>)
        n84 = property class="TabCtl"(reference=w176, "Value"=Main_Tabs_v0.1."Autocycle" ("Main Tab")) -> ()  [unwired: 1 in, 2 out]
      }
      frame "Autocycle Stats" {
        # "Parameters"
        n85 = Unbundle By Name(w183) -> ("Main Tab"=w182:refnum<vi>)
        n86 = property class="TabCtl"(reference=w182, "Value"=Main_Tabs_v0.1."Autocycle Statistics" ("Main Tab")) -> ()  [unwired: 1 in, 2 out]
      }
      frame "Autocycle IO" {
        # "Parameters"
        n87 = Unbundle By Name(w192) -> ("Main Tab"=w191:refnum<vi>)
        n88 = property class="TabCtl"(reference=w191, "Value"=Main_Tabs_v0.1."Autocycle IOs" ("Main Tab")) -> ()  [unwired: 1 in, 2 out]
        n89 = call-poly "Enqueue Message.vi"("error in (no error)"=w187, "Message"="Update IO", "Message Queue"=w185) -> ("error out"=w186:errorcluster)  [unwired: 7 in, 1 out]
      }
      frame "Update IO" {
        n90 = Unbundle By Name(w199) -> ("Main Tab"=w200:refnum<vi>)
        n91 = Wait (ms)(milliseconds to wait=u32 200) -> ()  [unwired: 1 out]
        n92 = property class="TabCtl"(reference=w200) -> ("Value"=w198:variant)  [unwired: 1 in, 2 out]
        n93 = Variant To Data(type=Main_Tabs_v0.1."Autocycle IOs" ("Main Tab"), Variant=w198) -> (data=w195:T4)  [unwired: 1 in, 1 out]
        n94 = global read "Maintenance GV.vi" "All IO"() -> (w204:T33)
        n95 = case shown="\"Autocycle IOs\"" w195 {
          tunnel: w202 -> [w212 w215]
          tunnel: [w212 w214] -> w201
          tunnel: w194 -> [_ w213]
          frame Default {
          }
          frame "Autocycle IOs" {
            n96 = call-poly "Enqueue Message.vi"("error in (no error)"=w215, "Message"="Update IO", "Message Queue"=w213) -> ("error out"=w214:errorcluster)  [unwired: 7 in, 1 out]
          }
        }
        n97 = Unbundle(w204) -> ("DI 1"=→"DI 1":T17, "DI 2"=→"DI 2":T34, "IAS 1"=→"IAS 1":dbl, "IAS 2"=→"IAS 2":dbl, "IAS 3"=→"IAS 3":dbl, "IAS 4"=→"IAS 4":dbl, "DO 1"=→"DO 1":T35)
      }
      frame "Update UI" {
        # "Update Display - Convert the message data to a string to display in the Data Display indicator."
        n98 = Variant To Data(error in=w231, type=T23 {"Array"=[], "Machine Status"=""} ("Status Cluster"), Variant=w230) -> (data=w226:T23, error out=w229:errorcluster)
        n99 = Unbundle(w226) -> ("Array"=→"Statuses":string[][], "Machine Status"=w224:string)
        "Status" <- w224
        n100 = Search and Replace String(input string=w224, search string="Autocycle is Running") -> (number of replacements=w222:i32)  [unwired: 6 in, 3 out]
        n101 = Greater Than 0?(x=w222) -> (x > 0?=w220:bool)
        n102 = Select(t=T22."Disabled and Grayed Out" ("Disabled"), s=w220, f=T22."Enabled" ("Disabled")) -> (s? t:f=w219:T22)
        n103 = property on="Home AC" class="Bool"("DisabledEnum"=w219) -> ()  [unwired: 2 in, 2 out]
        n104 = Merge Errors(w229) -> (w232:errorcluster)
      }
      frame "Autocycle Log" {
        # "Update Display - Convert the message data to a string to display in the Data Display indicator."
        n105 = Variant To Data(error in=w262, type=T25 {"Time-Stamp"=timestamp(0 s since 1904-01-01), "Auto Times"={"Index Time"=0, "TF Time"=0, "Insertion Time"=0, "Cutting Time"=0, "PF Time"=0, "Meas. Time"=0, "Reject Time"=0}, "Measurements"={"1"=0.0, "2"=0.0, "3"=0.0, "4"=0.0}, "Outputs"={"Good Parts"=0, "Reject Parts"=0}, "Cycle Time"=0.0, "Remarks"=""} ("Auto Stats"), Variant=w261) -> (data=w257:T25, error out=w260:errorcluster)
        n106 = Unbundle By Name(w257) -> ("Time-Stamp"=w255:timestamp, "Measurements"=w245:cluster{"1":dbl, "2":dbl, "3":dbl, "4":dbl}, "Outputs"=→"Output Chart":cluster{"Good Parts":u32, "Reject Parts":u32}, "Auto Times"=→"Auto Times":T9)
        "Latest Measure." <- w245
        n107 = call "Stats Unbundle.vi"("State"=Logging_FGV."Log Index", "Auto Stats"=w257) -> ("Cycle Time"=→"Cycle Time" →"Total Time":dbl, "Counters"=w250:cluster{"GoodCount":u32, "RejectCount":u32}, "OEE Cluster"=→"OEE Chart" →"OEE 2":T14, "Avg. Cycle Time"=→"Avg. Time":dbl, "Total Times"=→"Time Chart":T13)  [unwired: 4 in, 1 out]
        n108 = Unbundle By Name(w250) -> ("GoodCount"=w234:u32, "RejectCount"=w235:u32)
        "Rejects" <- w235
        "Good" <- w234
        "Good Count" <- w234
        "Reject Count" <- w235
        n109 = Unbundle(w245) -> ("1"=w244:dbl, "2"=w243:dbl, "3"=w242:dbl, "4"=w241:dbl)
        n110 = Add(x=w234, y=w235) -> (x+y=→"Total Count 2":u32)
        n111 = Bundle("1"=w244, "2"=w243, "3"=w242, "4"=w241, "4"=187.9, "4"=189.9) -> (→"Measurement Chart":T16)  [unwired: 1 in]
        n112 = Format Date/Time String(time format string (%c)="%d-%m-%Y | %H:%M:%S%3u", seconds (now)=w255) -> (date/time string=→"Timestamp":string)  [unwired: 1 in]
        n113 = Merge Errors(w260) -> (w263:errorcluster)
      }
      frame "Run Manual" {
        # "Update Manual mode"
        n114 = Bundle("Manual Para"="Manual Para", "Reject Pallets"="Reject Pallets") -> (w267:T36)  [unwired: 1 in]
        n115 = for {
          tunnel: w270 -> [w278] mode=indexing
          tunnel: T22."Disabled and Grayed Out" ("Disabled") -> [w277]
          n116 = property class="Bool"(reference=w278, "DisabledEnum"=w277) -> ()  [unwired: 1 in, 2 out]
        }
        n117 = call "Write NS (HMI).vi"("error in (no error)"=w273, "Message Data"=w267, "Message"="Manual Run") -> ("error out"=w272:errorcluster)  [unwired: 8 in]
        n118 = Merge Errors(w272) -> (w275:errorcluster)
      }
      frame "Manual Status" {
        n119 = Variant To Data(error in=w306, type=T26 {"Auto Times"={"Index Time"=0, "TF Time"=0, "Insertion Time"=0, "Cutting Time"=0, "PF Time"=0, "Meas. Time"=0, "Reject Time"=0}, "Results"={"Measurements"={"1"=0.0, "2"=0.0, "3"=0.0, "4"=0.0}, "Reject Pallets"={"Reject 1"=FALSE, "Reject 2"=FALSE, "Reject 3"=FALSE, "Reject 4"=FALSE}}, "OutputCount"=0, "error out"={"status"=FALSE, "code"=0, "source"=""}} ("cluster"), Variant=w305) -> (data=w302:T26, error out=w297:errorcluster)
        n120 = Unbundle(w302) -> ("Auto Times"=w301:T9, "Results"=w293:T37, "OutputCount"=w292:u32, "error out"=w295:errorcluster)
        n121 = for {
          tunnel: w303 -> [w312] mode=indexing
          tunnel: T22."Enabled" ("Disabled") -> [w311]
          n122 = property class="Bool"(reference=w312, "DisabledEnum"=w311) -> ()  [unwired: 1 in, 2 out]
        }
        n123 = Unbundle(w293) -> ("Measurements"=w281:cluster{"1":dbl, "2":dbl, "3":dbl, "4":dbl}, "Reject Pallets"=w282:T3)
        "Measurements" <- w281
        n124 = Bundle("Auto Times"=w301, "error out"=w295) -> (→"Status 2":T10)  [unwired: 1 in]
        n125 = Bundle("Reject Pallets"=w282, "Measurements"=w281) -> (w280:T38)  [unwired: 1 in]
        n126 = call "Counts Update (manual).vi"("output cluster"=w280, "Desired Cycle Time (s)"="Ideal Time", "AVL"="AVL", "OutputCount"=w292, "Counts in"=w296) -> ("OEE"=w286:T14, "Counts out"=w291:cluster{"OutputCount":u32, "RejectCount":u32})  [unwired: 5 in]
        n127 = Unbundle(w286) -> ("PRF"=→"PRF":dbl, "QUA"=→"QUA":dbl, "OEE"=→"OEE":dbl)  [unwired: 1 out]
        n128 = Unbundle(w291) -> ("OutputCount"=→"Output Count":u32, "RejectCount"=→"Rejects 2":u32)
        n129 = case shown="True" "Continuous?" {
          tunnel: w298 -> [_ w310]
          tunnel: w295 -> [_ w309]
          frame False {
          }
          frame True {
            # "Run if continuous is TRUE & No Error"
            n130 = call-poly "Enqueue Message.vi"("error in (no error)"=w309, "Message"="Run Manual", "Message Queue"=w310) -> ()  [unwired: 7 in, 2 out]
          }
        }
      }
      frame "Reset Manual Count" {
        w314 = u32 0 ("Rejects")
        n131 = local write "Rejects 2"(w314) -> ()
        n132 = local write "Output Count"(w314) -> ()
      }
      frame "Error" {
        w322 = 128  # call and forget
        # "Run async so that this loop will continue to run"
        # "Error"
        n133 = Variant To Data(error in=w341, type=errorcluster {"status"=FALSE, "code"=0, "source"=""} ("error constant"), Variant=w339) -> (data=w334:errorcluster, error out=w337:errorcluster)
        n134 = Unbundle By Name(w334) -> ("source"=w333:string)
        n135 = vi-ref "NewDialog.vi"() -> (w329:refnum<vi>)
        n136 = property class="VI"(reference=w329) -> (error out=w331:errorcluster, "Name"=w330:string)  [unwired: 1 in, 1 out]
        n137 = Search and Replace String(input string=w333, search string="<err>") -> (result string=w321:string)  [unwired: 6 in, 3 out]
        n138 = Open VI Reference(type specifier VI Refnum (for type only)=refnum<vi> refnum, vi path=w330, options=w322, error in (no error)=w331) -> (vi reference=w324:refnum<vi>, error out=w325:errorcluster)  [unwired: 2 in]
        n139 = call-by-ref "Start Asynchronous Call"(reference=w324, error in=w325, "inIcon"=T27."Error", "inTitle"="ERROR", "inMessage"=w321) -> (reference out=w327:refnum<vi>, error out=w326:errorcluster)  [unwired: 6 in, 3 out]
        n140 = Close Reference(reference=w327, error in (no error)=w326) -> (error out=w328:errorcluster)
        n141 = call <vilib>:"Simple Error Handler.vi"("error in (no error)"=w328) -> ()  [unwired: 4 in, 5 out]
        n142 = Merge Errors(w337) -> (w336:errorcluster)
      }
      frame "Confirm Quit" {
        # "Confirm Quit - Message that can confirm whether or not the user wants to exit the application."
        n143 = call "NewDialog.vi"("inIcon"=T27."Information", "inTitle"="SHUTDOWN?", "inButton2Text"="Shutdown", "inButton1Text"="", "inMessage"="Are you sure you want to shutdown?") -> ("outButton2"=w343:bool)  [unwired: 4 in, 2 out]
        "Shutdown?" <- w343
        n144 = case shown="True" w343 {
          tunnel: w354 -> [w355 w360]
          tunnel: [w355 w359] -> w351
          tunnel: w350 -> [_ w358]
          frame False {
          }
          frame True {
            n145 = call-poly "Enqueue Message.vi"("Priority Message? (F)"=TRUE, "error in (no error)"=w360, "Message"="Exit", "Message Queue"=w358) -> ("error out"=w359:errorcluster)  [unwired: 6 in, 1 out]
          }
        }
        n146 = Merge Errors(w351) -> (w352:errorcluster)
      }
      frame "Exit" {
        # "Stop the VI"
        # "Release the message queue reference"
        # "Exit - Exit the application."
        n147 = Variant To Data(type=errorcluster {"status"=FALSE, "code"=0, "source"=""} ("error constant"), Variant=w366) -> (data=w367:errorcluster)  [unwired: 1 in, 1 out]
        n148 = call <vilib>:"Simple Error Handler.vi"("error in (no error)"=w367) -> ()  [unwired: 4 in, 5 out]
        n149 = Send Notification(notification=TRUE, notifier=w365) -> (error out=w363:errorcluster)  [unwired: 1 in, 1 out]
        n150 = call "Fire User Event - Stop.vi"("User Event - Stop"=w371) -> ("error out"=w370:errorcluster)  [unwired: 10 in]
        n151 = Release Queue(queue=w376, error in (no error)=w369) -> (error out=w373:errorcluster)  [unwired: 1 in, 2 out]
        n152 = Merge Errors(w363, w370, w373) -> (w372:errorcluster)
      }
      frame Default {
        # "'Default' case only runs if there is a message that isn't defined in any of the other cases.  Output a programming error."
        n153 = xnode "Error Ring"("parameter 0"=w379) -> ("error out"=w380:errorcluster)
      }
    }
    n154 = call "Error Handler - Message Handling Loop.vi"("error in (no error)"=w54, "Message Queue"=w56) -> ("dup error in"=w55:errorcluster)  [unwired: 8 in, 1 out]
  }
  n155 = while {
    tunnel: w33 -> [w396]
    shift-right: [w394] -> w39
    shift-left: w36 -> [w395]
    tunnel: [w390] -> w37
    stop <- w392 stop-if-true
    # "Event Handling Loop"
    n156 = event shown="[9] \"End Cycle\", \"Enable Cutting?\", \"Enable TF?\", \"Enable PF?\", \"Enable Index?\", \"Enable Measure?\", \"Enable Reject?\", \"Enable Agitate?\", \"Enable BF?\", \"Enable Insertion?\": Value Change" {
      selector: w395 -> [_ _ _ _ _ _ _ _ _ _ _ _ _ _ _ _ _ _]
      dyn-events: [_ _ _ _ _ _ _ _ _ _ _ _ _ _ _ _ _ _] -> w394
      timeout: 500 -> [_ _ _ _ _ _ _ _ _ _ _ _ _ _ _ _ _ _]
      tunnel: [_ _ _ _ _ _ _ _ _ _ _ _ _ _ _ _ _ TRUE ("Discard?")] -> w392
      tunnel: w396 -> [w401 w405 w410 w414 w418 w422 w426 w431 w436 w441 w445 w450 w452 w455 w486 w495 w504 w506]
      tunnel: [w400 _ w409 w413 w417 w421 w425 w430 w435 w442 _ w448 w453 w458 _ _ _ _] -> w393
      tunnel: [w399 w405 w408 w412 w416 w420 w424 w429 w434 w441 w445 w449 w452 w454 w486 w495 w504 w506] -> w391
      event Panel Close? {
        n157 = event-data() -> ()  [unwired: 1 in, 1 out]
        n158 = call-poly "Enqueue Message.vi"("Priority Message? (F)"=TRUE, "Message"="Exit", "Message Queue"=w401) -> ("error out"=w400:errorcluster, "dup Message Queue"=w399:refnum<queue>)  [unwired: 7 in]
        n159 = event-data("Discard?"=TRUE) -> ()  [unwired: 1 in, 1 out]
      }
      event Timeout {
        n160 = event-data() -> ()  [unwired: 1 in, 1 out]
        n161 = Format Date/Time String(time format string (%c)="%d %b %Y | %I:%M:%S %p") -> (date/time string=→"Date-Time":string)  [unwired: 2 in]
      }
      event "Shutdown": Value Change {
        n162 = event-data() -> ()  [unwired: 1 in, 1 out]
        n163 = call-poly "Enqueue Message.vi"("Priority Message? (F)"=TRUE, "Message"="Confirm Quit", "Message Queue"=w410) -> ("error out"=w409:errorcluster, "dup Message Queue"=w408:refnum<queue>)  [unwired: 7 in]
      }
      event "Home Para", "Home Manual", "Home IOs": Value Change {
        n164 = event-data() -> ()  [unwired: 1 in, 1 out]
        n165 = call-poly "Enqueue Message.vi"("Message"="Initialize", "Message Queue"=w414) -> ("error out"=w413:errorcluster, "dup Message Queue"=w412:refnum<queue>)  [unwired: 8 in]
      }
      event "Back Stats", "Back IO": Value Change {
        n166 = event-data() -> ()  [unwired: 1 in, 1 out]
        n167 = call-poly "Enqueue Message.vi"("Message"="Autocycle Back", "Message Queue"=w418) -> ("error out"=w417:errorcluster, "dup Message Queue"=w416:refnum<queue>)  [unwired: 8 in]
      }
      event "Stats": Value Change {
        n168 = event-data() -> ()  [unwired: 1 in, 1 out]
        n169 = call-poly "Enqueue Message.vi"("Message"="Autocycle Stats", "Message Queue"=w422) -> ("error out"=w421:errorcluster, "dup Message Queue"=w420:refnum<queue>)  [unwired: 8 in]
      }
      event "All IO", "All IOs": Value Change {
        n170 = event-data() -> ()  [unwired: 1 in, 1 out]
        n171 = call-poly "Enqueue Message.vi"("Message"="Autocycle IO", "Message Queue"=w426) -> ("error out"=w425:errorcluster, "dup Message Queue"=w424:refnum<queue>)  [unwired: 8 in]
      }
      event "Home AC": Value Change {
        n172 = event-data() -> ()  [unwired: 1 in, 1 out]
        n173 = call-poly "Enqueue Message.vi"("Message"="Initialize", "Message Queue"=w431) -> ("error out"=w430:errorcluster, "dup Message Queue"=w429:refnum<queue>)  [unwired: 8 in]
        n174 = call "Write NS (HMI).vi"("Message"="Exit Autocycle") -> ()  [unwired: 10 in, 1 out]
      }
      event "Maintenance", "Parameters", "Manual": Value Change {
        n175 = event-data() -> ("CtlRef"=w433:refnum<vi>)  [unwired: 1 in]
        n176 = property class="Bool"(reference=w433) -> ("Label.Text"=w432:string)  [unwired: 1 in, 2 out]
        n177 = call-poly "Enqueue Message.vi"("Message"=w432, "Message Queue"=w436) -> ("error out"=w435:errorcluster, "dup Message Queue"=w434:refnum<queue>)  [unwired: 8 in]
      }
      event "End Cycle", "Enable Cutting?", "Enable TF?", "Enable PF?", "Enable Index?", "Enable Measure?", "Enable Reject?", "Enable Agitate?", "Enable BF?", "Enable Insertion?": Value Change {
        n178 = event-data() -> ("CtlRef"=w443:refnum<vi>, "NewVal"=w437:bool)  [unwired: 1 in, 1 out]
        n179 = property class="Bool"(reference=w443) -> ("Label.Text"=w440:string)  [unwired: 1 in, 2 out]
        n180 = Concatenate Strings("GV:" ("string"), w440) -> (w438:string)
        n181 = call "Write NS (HMI).vi"("Message Data"=w437, "Message"=w438) -> ("error out"=w442:errorcluster)  [unwired: 9 in]
      }
      event "Reset MCount": Value Change {
        n182 = event-data() -> ()  [unwired: 1 in, 6 out]
        n183 = call-poly "Enqueue Message.vi"("Message"="Reset Manual Count", "Message Queue"=w445) -> ()  [unwired: 8 in, 2 out]
      }
      event "Run Manual": Value Change {
        n184 = event-data() -> ("CtlRef"=w447:refnum<vi>)  [unwired: 1 in, 2 out]
        n185 = property class="Bool"(reference=w447) -> ("Label.Text"=w446:string)  [unwired: 1 in, 2 out]
        n186 = call-poly "Enqueue Message.vi"("Message"=w446, "Message Queue"=w450) -> ("error out"=w448:errorcluster, "dup Message Queue"=w449:refnum<queue>)  [unwired: 8 in]
      }
      event "Toggle Motor": Value Change {
        n187 = event-data() -> ()  [unwired: 1 in, 3 out]
        n188 = call "Write NS (HMI).vi"("Message"="Toggle Motor") -> ("error out"=w453:errorcluster)  [unwired: 10 in]
      }
      event "Save Para": Value Change {
        n189 = event-data() -> ()  [unwired: 1 in, 3 out]
        n190 = Cluster To Array(cluster="Agitator Para") -> (array=w475:u32[])
        n191 = Cluster To Array(cluster="Tube Feeder Para") -> (array=w473:u32[])
        n192 = Cluster To Array(cluster="Insertion Para") -> (array=w471:u32[])
        n193 = Cluster To Array(cluster="Cutting Para") -> (array=w469:u32[])
        n194 = Cluster To Array(cluster="PF Para") -> (array=w467:u32[])
        n195 = Cluster To Array(cluster="Meas. Para") -> (array=w465:dbl[])
        n196 = Cluster To Array(cluster="Reject Para") -> (array=w463:u32[])
        n197 = Cluster To Array(cluster="BF Para") -> (array=w461:u32[])
        n198 = Bundle By Name(cluster=T2 {"Agitator Delays"=[1000], "TF Delays"=[1000], "Insertion Delays"=[1000], "Cutting Delays"=[1000], "PF Delays"=[1000], "Measur. Delays"=[1000.0], "Reject Delays"=[1000], "BF Delays"=[1000]} ("Auto Para"), "Agitator Delays"=w475, "TF Delays"=w473, "Insertion Delays"=w471, "Cutting Delays"=w469, "PF Delays"=w467, "Measur. Delays"=w465, "Reject Delays"=w463, "BF Delays"=w461) -> (w460:T2)
        n199 = Bundle("Auto Para"=w460, "General Para"="General Para") -> (w457:cluster{"Auto Para":T2, "General Para":T1})  [unwired: 1 in]
        n200 = property on="Auto Para" class="Clust (strict)"("Value"=w460) -> ()  [unwired: 2 in, 2 out]
        n201 = call-poly "Enqueue Message.vi"("Message Data"=w457, "Message"="Update Para", "Message Queue"=w455) -> ("error out"=w458:errorcluster, "dup Message Queue"=w454:refnum<queue>)  [unwired: 7 in]
      }
      event "Insertion Para.Delay 1", "Insertion Para.Delay 2", "Agitator Para.Delay", "Agitator Para.Timeout", "Cutting Para.Delay", "Cutting Para.Delay 2", "Cutting Para.Delay 3", "Tube Feeder Para.Delay", "Tube Feeder Para.Delay 2", "Tube Feeder Para.Max Attempts", "PF Para.Delay", "PF Para.Timeout", "Reject Para.Delay", "BF Para.Delay 1", "BF Para.Delay 2": Mouse Up {
        n202 = event-data() -> ("CtlRef"=w478:refnum<vi>)  [unwired: 1 in, 4 out]
        n203 = property class="DigNum (strict)"(reference=w478) -> (reference out=w481:refnum<vi>, "Value"=w482:u32)  [unwired: 1 in, 1 out]
        n204 = Number To Fractional String(number=w482, precision (6)=0.0 ("width (-)")) -> (F-format string=w480:string)  [unwired: 2 in]
        n205 = call "HMI Pop Up Num KP v1.1.vi"("String In"=w480) -> ("String Out"=w479:string)  [unwired: 9 in, 1 out]
        n206 = Fract/Exp String To Number(string=w479, default (0 dbl)=0.0 ("default (0 I32)")) -> (number=w484:dbl)  [unwired: 2 in, 1 out]
        n207 = property class="DigNum (strict)"(reference=w481, "Value"=w484) -> ()  [unwired: 1 in, 2 out]
      }
      event "Meas. Para.Delay": Mouse Up {
        n208 = event-data() -> ("CtlRef"=w487:refnum<vi>)  [unwired: 1 in, 4 out]
        n209 = property class="DigNum (strict)"(reference=w487) -> (reference out=w490:refnum<vi>, "Value"=w491:dbl)  [unwired: 1 in, 1 out]
        n210 = Number To Fractional String(number=w491, precision (6)=0.0 ("width (-)")) -> (F-format string=w489:string)  [unwired: 2 in]
        n211 = call "HMI Pop Up Num KP v1.1.vi"("String In"=w489) -> ("String Out"=w488:string)  [unwired: 9 in, 1 out]
        n212 = Fract/Exp String To Number(string=w488, default (0 dbl)=0.0 ("default (0 I32)")) -> (number=w493:dbl)  [unwired: 2 in, 1 out]
        n213 = property class="DigNum (strict)"(reference=w490, "Value"=w493) -> ()  [unwired: 1 in, 2 out]
      }
      event "Meas. Para.Mean Length", "Meas. Para.Tolerance": Mouse Up {
        n214 = event-data() -> ("CtlRef"=w496:refnum<vi>)  [unwired: 1 in, 4 out]
        n215 = property class="DigNum (strict)"(reference=w496) -> (reference out=w499:refnum<vi>, "Value"=w500:dbl)  [unwired: 1 in, 1 out]
        n216 = Number To Fractional String(number=w500, precision (6)=2.0 ("width (-)")) -> (F-format string=w498:string)  [unwired: 2 in]
        n217 = call "HMI Pop Up Num KP v1.1.vi"("String In"=w498) -> ("String Out"=w497:string)  [unwired: 9 in, 1 out]
        n218 = Fract/Exp String To Number(string=w497, default (0 dbl)=0.0 ("default (0 I32)")) -> (number=w502:dbl)  [unwired: 2 in, 1 out]
        n219 = property class="DigNum (strict)"(reference=w499, "Value"=w502) -> ()  [unwired: 1 in, 2 out]
      }
      event User Event {
        # "The Message Handling Loop processed an \"Exit\" message, which fired this event to stop the Event Handling Loop."
        n220 = event-data() -> ()  [unwired: 1 in, 1 out]
      }
    }
    n221 = call "Error Handler - Event Handling Loop.vi"("error in (no error)"=w393, "Message Queue"=w391) -> ("dup error in"=w390:errorcluster)  [unwired: 8 in, 1 out]
  }
  n222 = call "HMI-cRIO Connection Manager.vi"("error in"=w5, "notifier in"=w6, "Queue in"=w33) -> ("error out"=w27:errorcluster, "Notifier out"=w28:refnum<notifier>)  [unwired: 7 in]
  n223 = Unregister For Events(event registration refnum=w39, error in=w37) -> (error out=w40:errorcluster)
  n224 = Merge Errors(w40, w42, w27) -> (w41:errorcluster)
  n225 = call "Destroy User Event - Stop.vi"("error in (no error)"=w41, "User Event - Stop"=w35) -> ("error out"=w30:errorcluster)  [unwired: 9 in]
  n226 = Release Notifier(notifier=w28, error in (no error)=w30) -> (error out=w29:errorcluster)  [unwired: 1 in, 2 out]
  n227 = disable-structure shown="RUN_TIME_ENGINE==True" {
    disable-tunnel: w29 -> [_ _]
    frame condition #0 (active) {
    }
    frame condition #1 {
      n228 = local read "Shutdown?"() -> (w507:bool)
      n229 = case shown="True" w507 {
        tunnel: [_ w509] -> w508
        frame False {
        }
        frame True {
          n230 = call <vilib>:"System Exec.vi"("wait until completion? (T)"=TRUE, "command line"="Shutdown -s -f -t 10") -> ("error out"=w509:errorcluster)  [unwired: 6 in, 3 out]
        }
      }
      n231 = flat-sequence {
        tunnel: w508 -> [_]
        frame #0 {
          n232 = Quit LabVIEW() -> ()  [unwired: 1 in]
        }
      }
    }
  }
